vi "Status.vi"(8 "error in (no error)":errorcluster, 11 "Name":string) -> (0 "error out":errorcluster, 1 "Start?":bool, 2 "TimePeroid(ms)":i64, 3 "Exist?":bool, 4 "EclipsedTime(ms)":i64)   [LabVIEW 2017, in "TimerEngine.lvlib" / "TimerEngine.lvclass"]
uses:
  TimerEngine.lvclass
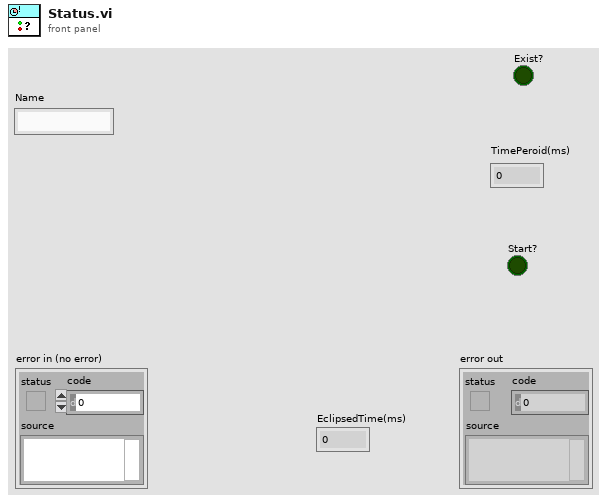
[diagram p1: front panel]
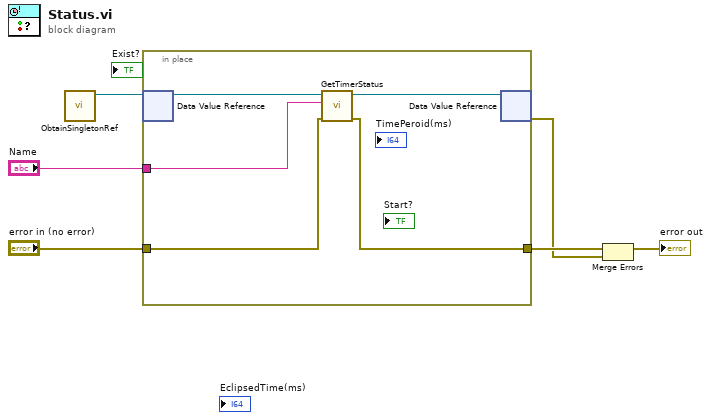
[diagram p0: block diagram]
diagram:
  n1 = call "ObtainSingletonRef.vi"() -> ("data value reference"=w6:refnum<data-value>)  [unwired: 10 in, 1 out]
  n2 = in-place {
    in-place-border: [w7] -> w5
    in-place-border: "error in (no error)" -> [w9]
    in-place-border: "Name" -> [w8]
    n3 = in-place-dvr #1(w6) -> (w11:refnum<class "TimerEngine.lvclass">)  [unwired: 1 out]
    n4 = call "GetTimerStatus.vi"("error in (no error)"=w9, "Name"=w8, "TimerEngine in"=w11) -> ("error out"=w7:errorcluster, "TimerEngine out"=w10:refnum<class "TimerEngine.lvclass">)  [unwired: 3 in, 4 out]
    n5 = in-place-dvr #1(w10) -> (w2:errorcluster)  [unwired: 1 out]
  }
  n6 = Merge Errors(w5, w2) -> (→"error out":errorcluster)
